vi "GetLimits.vi"(8 "error in (no error)":errorcluster, 11 "Stage_MadCityLab in":refnum<class "Stage_MadCityLab.lvclass">) -> (0 "error out":errorcluster, 2 "Limits":cluster{"Upper limit":dbl, "Lower limit":dbl}[](array[cluster]), 3 "Stage_MadCityLab out":refnum<class "Stage_MadCityLab.lvclass">)   [LabVIEW 2020, in "Stage_MadCityLab.lvlib" / "Stage_MadCityLab.lvclass"]
uses:
  Stage_MadCityLab.lvclass
  Hardware Abstraction Layer/Component/Stage/Stage/Stage.lvclass
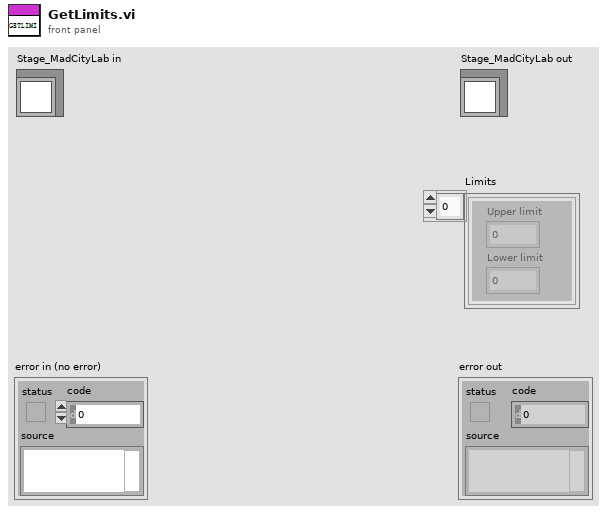
[diagram p1: front panel]
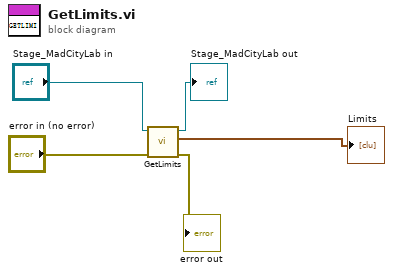
[diagram p0: block diagram]
diagram:
  n1 = call-parent "GetLimits.vi"("error in (no error)"="error in (no error)", "Stage in"="Stage_MadCityLab in") -> ("error out"=→"error out":errorcluster, "Limits"=→"Limits":cluster{"Upper limit":dbl, "Lower limit":dbl}[], "Stage out"=→"Stage_MadCityLab out":refnum<class "Stage_MadCityLab.lvclass">)  [unwired: 7 in]
